vi "Create MM Cluster.vi"(8 "error out":errorcluster, 11 "Channel Refs":T4[](array[typedef]) format="%.0x") -> (0 "error out 2":errorcluster, 3 "MM Data":T1)   [LabVIEW 2018, in "Vires VTD System Explorer.lvlib"]
uses:
  Vires VTD System Explorer.lvlib
  <vilib>/NI Veristand/Custom Device API/Custom Device Item Ref.ctl
  MM/MM Data.ctl
  MM/MM Objects.ctl
  MM/MM Object.ctl
  <vilib>/NI Veristand/Custom Device API/Get Item Property (Variant).vi
  <vilib>/NI Veristand/Custom Device API/Custom Device API.lvlib
  MM/MM.lvlib
  Shared/Vires VTD Shared.lvlib
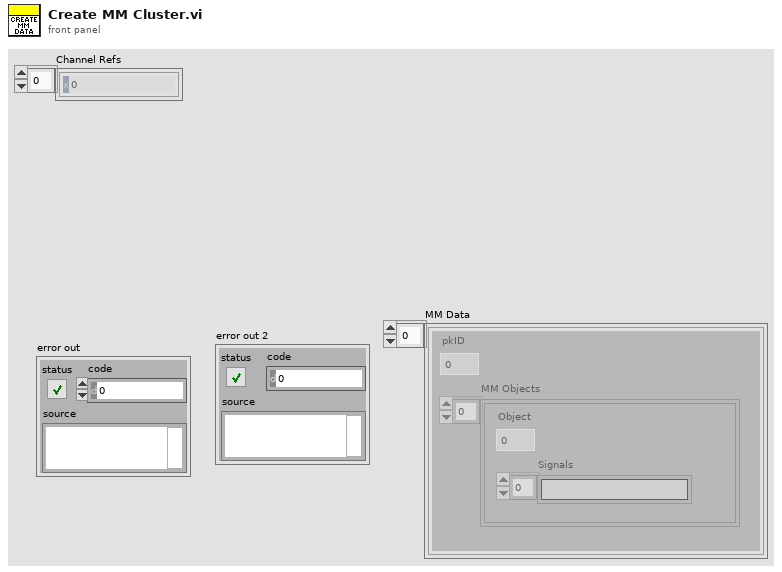
[diagram p1: front panel]
types:
  T1 = typedef "Vires VTD Shared.lvlib/MM Data.ctl" = T2[]
  T2 = typedef "MM.lvlib/MM Objects.ctl" = cluster{"pkID":i32, "MM Objects":T3[]}
  T3 = typedef "MM.lvlib/MM Object.ctl" = cluster{"Object":i32, "Signals":string[]}
  T4 = typedef "Custom Device API.lvlib/Custom Device Item Ref.ctl" = u64
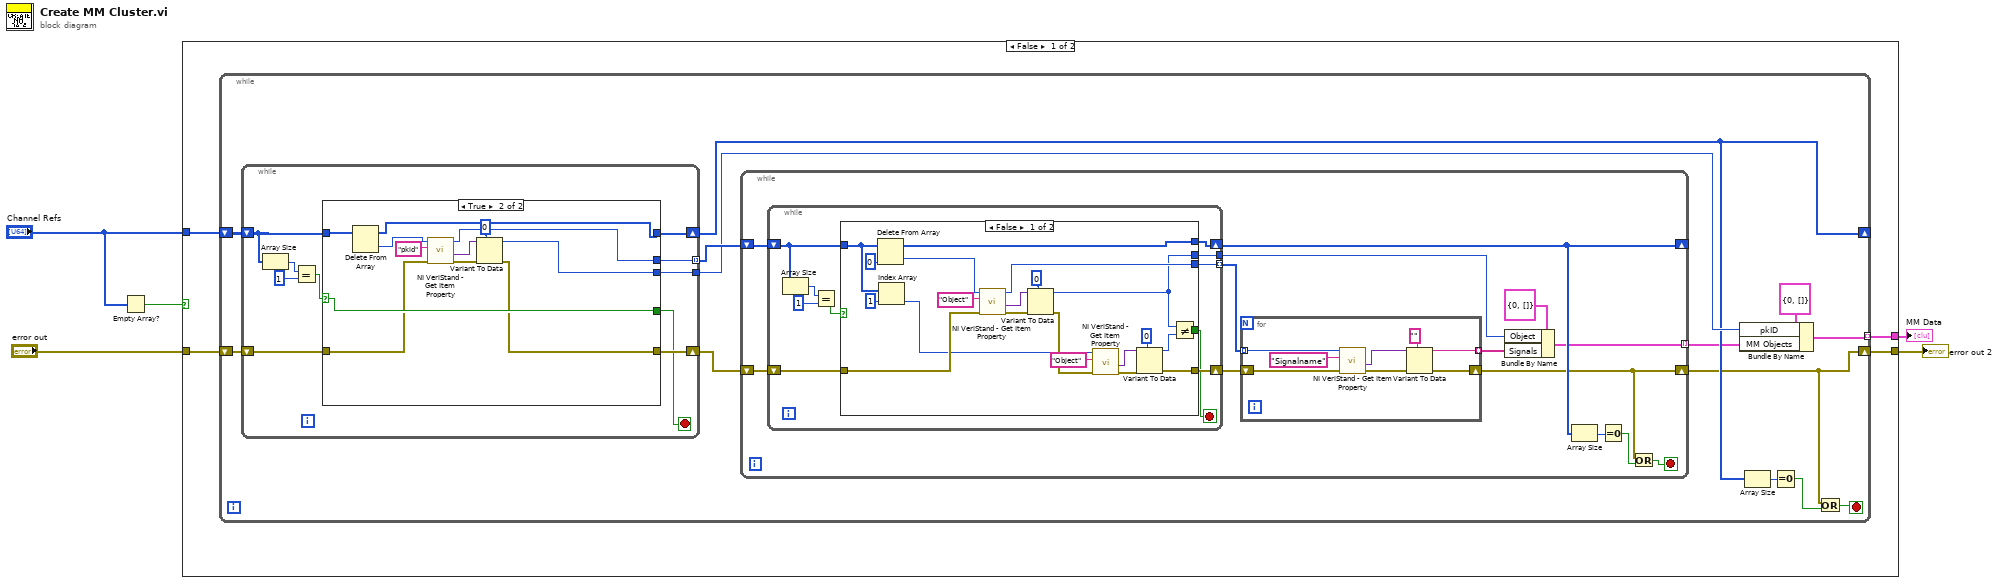
[diagram p0: block diagram]
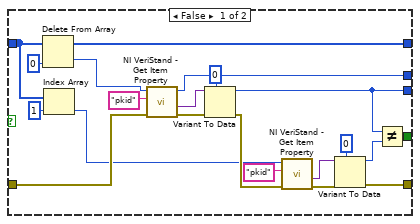
[diagram p2: hidden frame]
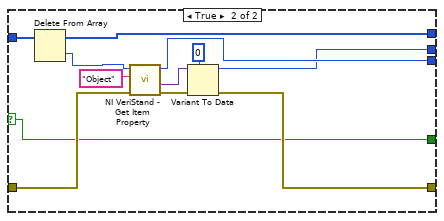
[diagram p3: hidden frame]
diagram:
  n1 = Empty Array?(array="Channel Refs") -> (empty?=w2:bool)
  n2 = case shown="False" w2 {
    tunnel: "Channel Refs" -> [w9 _]
    tunnel: "error out" -> [w8 w130]
    tunnel: [w7 w130] -> w4
    tunnel: [w6 _] -> w1
    frame False {
      n3 = while {
        shift-right: [w14] -> _
        shift-left: w9 -> [w22]
        shift-right: [w13] -> w7
        shift-left: w8 -> [w18]
        tunnel: [w12] -> w6 mode=indexing
        stop <- w15 stop-if-true
        n4 = while {
          shift-right: [w32] -> w21
          shift-left: w18 -> [w31]
          tunnel: [w29] -> w20 mode=indexing
          tunnel: [w28] -> w19
          shift-right: [w27] -> w14
          shift-left: w22 -> [w26]
          stop <- w30 stop-if-true
          n5 = Array Size(array=w26) -> (size(s)=w25:i32)
          n6 = Equal?(x=w25, y=1) -> (x = y?=w23:bool)
          n7 = case shown="True" w23 {
            selector: w23 -> [_ w65]
            tunnel: [w46 w58] -> w32
            tunnel: w31 -> [w45 w59]
            tunnel: [w41 w65] -> w30
            tunnel: [w40 w56] -> w29
            tunnel: [w39 w57] -> w28
            tunnel: [w35 w54] -> w27
            tunnel: w26 -> [w33 w55]
            frame False {
              n8 = Delete From Array(array=w33, index=0) -> (deleted portion=w36:T4, array with subset deleted=w35:T4[])  [unwired: 1 in]
              n9 = Index Array(array=w33, index=1) -> (element=w34:T4)
              n10 = call-poly <vilib>:"NI VeriStand - Get Item Property.vi"("error in (no error)"=w45, "Property Name"="pkid", "Item Ref in"=w36) -> ("error out"=w51:errorcluster, "Value"=w50:variant, "Item Ref out"=w40:T4)  [unwired: 5 in, 1 out]
              n11 = Variant To Data(error in=w51, type=u8 0, Variant=w50) -> (data=w39:u8, error out=w49:errorcluster)
              n12 = call-poly <vilib>:"NI VeriStand - Get Item Property.vi"("error in (no error)"=w49, "Property Name"="pkid", "Item Ref in"=w34) -> ("error out"=w48:errorcluster, "Value"=w47:variant)  [unwired: 5 in, 2 out]
              n13 = Variant To Data(error in=w48, type=u8 0, Variant=w47) -> (data=w43:u8, error out=w46:errorcluster)
              n14 = Not Equal?(x=w39, y=w43) -> (x != y?=w41:bool)
            }
            frame True {
              n15 = Delete From Array(array=w55) -> (deleted portion=w60:T4, array with subset deleted=w54:T4[])  [unwired: 2 in]
              n16 = call-poly <vilib>:"NI VeriStand - Get Item Property.vi"("error in (no error)"=w59, "Property Name"="pkid", "Item Ref in"=w60) -> ("error out"=w63:errorcluster, "Value"=w62:variant, "Item Ref out"=w56:T4)  [unwired: 5 in, 1 out]
              n17 = Variant To Data(error in=w63, type=u8 0, Variant=w62) -> (data=w57:u8, error out=w58:errorcluster)
            }
          }
        }
        n18 = while {
          shift-right: [w72] -> _
          shift-left: w20 -> [w77]
          shift-right: [w68] -> w13
          shift-left: w21 -> [w78]
          tunnel: [w67] -> w10 mode=indexing
          stop <- w71 stop-if-true
          n19 = while {
            shift-right: [w88] -> w75
            shift-left: w78 -> [w87]
            tunnel: [w85] -> w76 mode=indexing
            tunnel: [w84] -> w73
            shift-right: [w79] -> w72
            shift-left: w77 -> [w81]
            stop <- w86 stop-if-true
            n20 = Array Size(array=w81) -> (size(s)=w82:i32)
            n21 = Equal?(x=w82, y=1) -> (x = y?=w80:bool)
            n22 = case shown="False" w80 {
              selector: w80 -> [_ w115]
              tunnel: [w102 w116] -> w88
              tunnel: w87 -> [w101 w117]
              tunnel: [w97 w115] -> w86
              tunnel: [w96 w114] -> w85
              tunnel: [w95 w113] -> w84
              tunnel: w81 -> [w94 w112]
              tunnel: [w89 w111] -> w79
              frame False {
                n23 = Delete From Array(array=w94, index=0) -> (deleted portion=w90:T4, array with subset deleted=w89:T4[])  [unwired: 1 in]
                n24 = Index Array(array=w94, index=1) -> (element=w93:T4)
                n25 = call-poly <vilib>:"NI VeriStand - Get Item Property.vi"("error in (no error)"=w101, "Property Name"="Object", "Item Ref in"=w90) -> ("error out"=w107:errorcluster, "Value"=w106:variant, "Item Ref out"=w96:T4)  [unwired: 5 in, 1 out]
                n26 = Variant To Data(error in=w107, type=u8 0, Variant=w106) -> (data=w95:u8, error out=w105:errorcluster)
                n27 = call-poly <vilib>:"NI VeriStand - Get Item Property.vi"("error in (no error)"=w105, "Property Name"="Object", "Item Ref in"=w93) -> ("error out"=w104:errorcluster, "Value"=w103:variant)  [unwired: 5 in, 2 out]
                n28 = Variant To Data(error in=w104, type=u8 0, Variant=w103) -> (data=w99:u8, error out=w102:errorcluster)
                n29 = Not Equal?(x=w95, y=w99) -> (x != y?=w97:bool)
              }
              frame True {
                n30 = Delete From Array(array=w112) -> (deleted portion=w110:T4, array with subset deleted=w111:T4[])  [unwired: 2 in]
                n31 = call-poly <vilib>:"NI VeriStand - Get Item Property.vi"("error in (no error)"=w117, "Property Name"="Object", "Item Ref in"=w110) -> ("error out"=w119:errorcluster, "Value"=w120:variant, "Item Ref out"=w114:T4)  [unwired: 5 in, 1 out]
                n32 = Variant To Data(error in=w119, type=u8 0, Variant=w120) -> (data=w113:u8, error out=w116:errorcluster)
              }
            }
          }
          n33 = for {
            tunnel: w76 -> [w127] mode=indexing
            shift-right: [w125] -> w68
            shift-left: w75 -> [w128]
            tunnel: [w122] -> w74 mode=indexing
            n34 = call-poly <vilib>:"NI VeriStand - Get Item Property.vi"("error in (no error)"=w128, "Property Name"="Signalname", "Item Ref in"=w127) -> ("error out"=w124:errorcluster, "Value"=w123:variant)  [unwired: 5 in, 2 out]
            n35 = Variant To Data(error in=w124, type="" ("Property Name"), Variant=w123) -> (data=w122:string, error out=w125:errorcluster)
          }
          n36 = Bundle By Name(cluster=T3 {"Object"=0, "Signals"=[]} ("RDB Player Object"), "Object"=w73, "Signals"=w74) -> (w67:T3)
          n37 = Array Size(array=w72) -> (size(s)=w70:i32)
          n38 = Equal To 0?(x=w70) -> (x = 0?=w69:bool)
          n39 = Or(x=w68, y=w69) -> (x .or. y?=w71:bool)
        }
        n40 = Bundle By Name(cluster=T2 {"pkID"=0, "MM Objects"=[]} ("MM Objects"), "pkID"=w19, "MM Objects"=w10) -> (w12:T2)
        n41 = Array Size(array=w14) -> (size(s)=w16:i32)
        n42 = Equal To 0?(x=w16) -> (x = 0?=w17:bool)
        n43 = Or(x=w13, y=w17) -> (x .or. y?=w15:bool)
      }
    }
    frame True {
    }
  }
  "error out 2" <- w4
  "MM Data" <- w1
